vi "test_LEDS_FPGA.vi"() -> ()   [LabVIEW 2015]
uses:
  <vilib>/rvi/Emulation/niFpgaGetClockAttributes.vi
  <vilib>/rvi/Emulation/niFpgaSctlEmulationGetInTimedLoop.vi
  <vilib>/rvi/Emulation/niFpgaEmulationReportErrorSimple.vi
  <vilib>/rvi/eio/common/nirviEmuTemplateMethod_errors.vi
  <vilib>/rvi/Emulation/niFpgaCriticalErrorInLSC.vi
  <vilib>/eio/EIONode/EIONode.xnode
panel:
  out "Boolean":bool
  in  "LED 2":bool
  in  "LED 1":bool
  in  "LED 0":bool
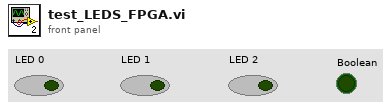
[diagram p1: front panel]
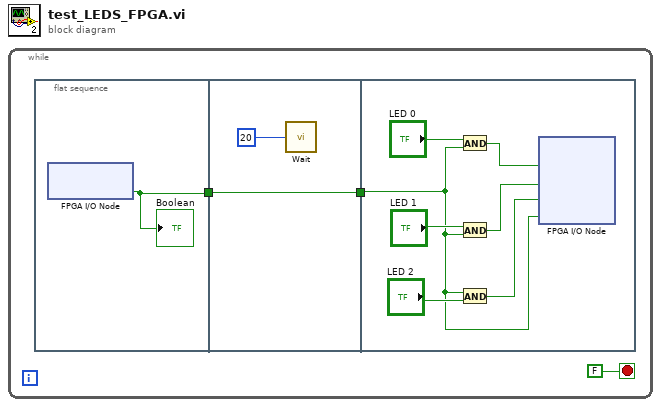
[diagram p0: block diagram]
diagram:
  n1 = while {
    stop <- FALSE stop-if-true
    n2 = flat-sequence {
      tunnel: [w4] -> w1
      tunnel: [w5] -> w2
      tunnel: w1 -> [w5]
      tunnel: w2 -> [w7]
      frame #0 {
        n3 = xnode "FPGA I/O Node"() -> ("Button0"=w4:bool)  [unwired: 1 in, 1 out]
        "Boolean" <- w4
      }
      frame #1 {
        n4 = call "Wait"("Count(Ticks)"=u32 20) -> ()  [unwired: 1 out]
      }
      frame #2 {
        n5 = And(x="LED 0", y=w7) -> (x .and. y?=w12:bool)
        n6 = And(x="LED 1", y=w7) -> (x .and. y?=w11:bool)
        n7 = And(x=w7, y="LED 2") -> (x .and. y?=w10:bool)
        n8 = xnode "FPGA I/O Node"("LED0"=w12, "LED1"=w11, "LED2"=w10, "LED3"=w7) -> ()  [unwired: 4 in, 4 out]
      }
    }
  }
